vi "SST.vi"(0 "System no.":i32=1 min=1 max=4 step=1, 2 "Axes to set":string[](array[string]), 3 "Step size":dbl[](array[numeric]) format="%.6f", 4 "No.of digits":i16=4, 5 "error in":errorcluster) -> (19 "error out":errorcluster)   [LabVIEW 2020]
doc: "Sets step size for manual control. No. of digits is the number of digits after the decimal point in the step size values that will be sent.\n\nC-702: Sets step size for cursor control (see also SCA.vi).\n\nC-848: Sets step size for cursor control (see also SCA.vi) and position control with a joystick connected to the C-848 (see also JEN.vi). \n\nC-867: Step size is applied to a motion caused by an Human Interface (HI) device. HI control must be configured appropriately with HIA (Function = 2 (relative position), DeviceAxis = 3 or 4). \n\nC-880: Sets step size for Manual Control Pad, cursor control (see also SCA.vi) and position control with a joystick connected to the C-880 (see also JEN.vi).\n\nE-871, E-873: Step size is applied to a motion caused by an Human Interface (HI) device. HI control must be configured appropriately with HIA (Function = 2 (relative position), DeviceAxis = 3 or 4)\n\nC-887, F-206, M-8X0: Sets step size for Manual Control Pad. Only axes X,Y,Z,U,V,W allowed."
panel:
  # "Sets stepsize for manual control."
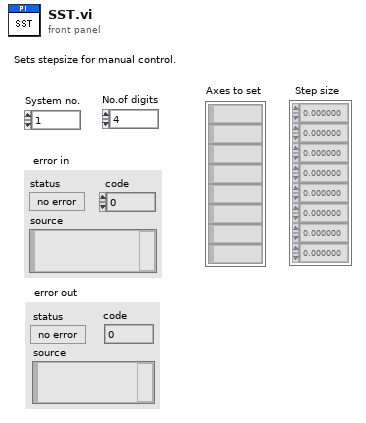
[diagram p1: front panel]
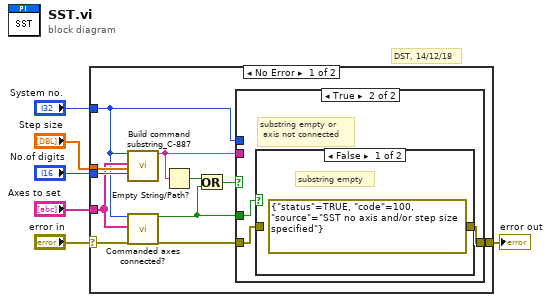
[diagram p0: block diagram]
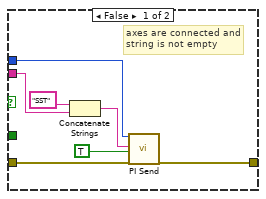
[diagram p2: hidden frame]
diagram:
  # "DST, 14/12/18"
  n1 = case shown="No Error" "error in" {
    selector: "error in" -> [w10 w30]
    tunnel: [w17 w30] -> w6
    tunnel: "Step size" -> [w16 _]
    tunnel: "No.of digits" -> [w15 _]
    tunnel: "System no." -> [w11 _]
    tunnel: "Axes to set" -> [w13 _]
    frame No Error {
      n2 = call "Build command substring_C-887.vi"("System no."=w11, "Affected axes"=w13, "Parameters"=w16, "No. of digits"=w15) -> ("Command substring"=w8:string)  [unwired: 3 in, 12 out]
      n3 = call "Commanded axes connected?.vi"("System no."=w11, "Commanded axes"=w13, "error in"=w10) -> ("Controller error"=w9:bool, "error out"=w14:errorcluster)  [unwired: 1 in, 14 out]
      n4 = Empty String/Path?(string/path=w8) -> (empty?=w7:bool)
      n5 = Or(x=w7, y=w9) -> (x .or. y?=w12:bool)
      n6 = case shown="True" w12 {
        tunnel: w8 -> [w23 _]
        tunnel: [w19 w27] -> w17
        tunnel: w14 -> [w20 w26]
        tunnel: w9 -> [_ w25]
        tunnel: w11 -> [w18 _]
        frame False {
          # "axes are connected and\nstring is not empty"
          n7 = Concatenate Strings("SST", w23) -> (w21:string)
          n8 = call "PI Send.vi"("System no."=w18, "String to send"=w21, "Attach termination char.?"=TRUE ("Attach Linefeed?"), "error in"=w20) -> ("error out"=w19:errorcluster)  [unwired: 2 in, 13 out]
        }
        frame True {
          # "substring empty or\n axis not connected"
          n9 = case shown="False" w25 {
            tunnel: [errorcluster {"status"=TRUE, "code"=100, "source"="SST no axis and/or step size specified"} ("error out") w29] -> w27
            tunnel: w26 -> [_ w29]
            frame False {
              # "substring empty"
            }
            frame True {
              # "commanded axis\nnot connected"
            }
          }
        }
      }
    }
    frame Error {
    }
  }
  "error out" <- w6
